vi "Create Files Directory.vi"(8 "error in (no error)":errorcluster, 11 "Setup File in":refnum<class "Setup File.lvclass">) -> (0 "error out":errorcluster, 3 "Setup File out":refnum<class "Setup File.lvclass">)   [LabVIEW 2012, in "Setup File.lvclass"]
uses:
  Setup File.lvclass
  Setup File.lvclass/Setup File.ctl
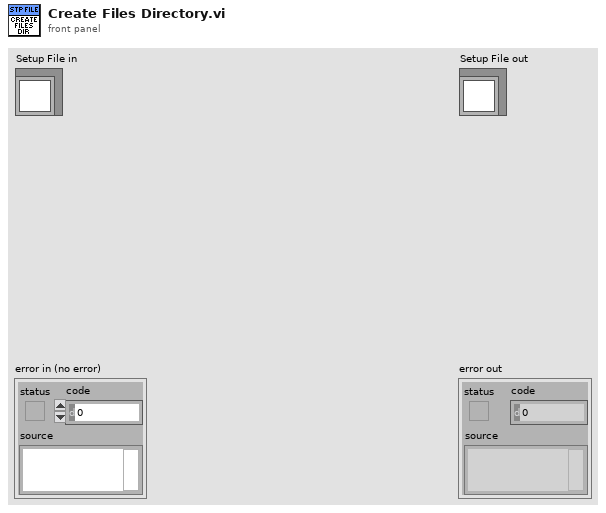
[diagram p1: front panel]
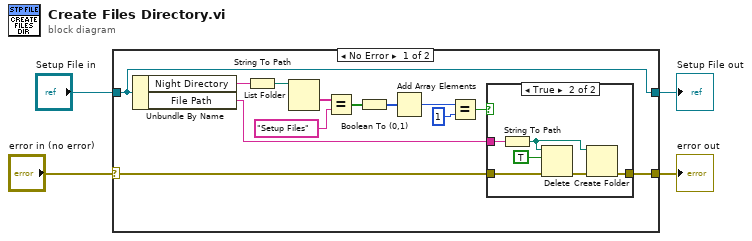
[diagram p0: block diagram]
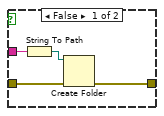
[diagram p2: hidden frame]
diagram:
  n1 = case shown="No Error" "error in (no error)" {
    selector: "error in (no error)" -> [w8 w29]
    tunnel: [w9 w29] -> w3
    tunnel: [w7 w28] -> w1
    tunnel: "Setup File in" -> [w7 w28]
    frame No Error {
      n2 = Unbundle By Name(w7) -> ("Night Directory"=w6:string, "File Path"=w5:string)
      n3 = String To Path(string=w6) -> (path=w17:path)
      n4 = List Folder(path=w17) -> (folder names=w16:string[])  [unwired: 3 in, 3 out]
      n5 = Equal?(x=w16, y="Setup Files") -> (x = y?=w12:bool[])
      n6 = Boolean To (0,1)(Boolean=w12) -> (0, 1=w13:i16[])
      n7 = Add Array Elements(numeric array=w13) -> (sum=w14:i16)
      n8 = Equal?(x=w14, y=i16 1) -> (x = y?=w11:bool)
      n9 = case shown="True" w11 {
        tunnel: [w20 w23] -> w9
        tunnel: w8 -> [w19 w27]
        tunnel: w5 -> [w18 w26]
        frame False {
          n10 = String To Path(string=w18) -> (path=w21:path)
          n11 = Create Folder(path (use dialog)=w21, error in=w19) -> (error out=w20:errorcluster)  [unwired: 1 in, 2 out]
        }
        frame True {
          n12 = String To Path(string=w26) -> (path=w22:path)
          n13 = Delete(path (use dialog)=w22, entire hierarchy (F)=TRUE, error in=w27) -> (error out=w24:errorcluster)  [unwired: 2 in, 2 out]
          n14 = Create Folder(path (use dialog)=w22, error in=w24) -> (error out=w23:errorcluster)  [unwired: 1 in, 2 out]
        }
      }
    }
    frame Error {
    }
  }
  "error out" <- w3
  "Setup File out" <- w1
